vi "get_name.vi"(0 "HGF_Reference":refnum<class "HGF_Reference.lvclass">, 5 "error in (no error)":errorcluster) -> (14 "dup HGF_Reference":refnum<class "HGF_Reference.lvclass">, 16 "name":string, 19 "error out":errorcluster)   [LabVIEW 2014, in "HGF_BaseClasses.lvlib" / "HGF_Reference.lvclass"]
doc: "Get name of this reference."
uses:
  HGF_Reference.lvclass
  HGF_Reference.lvclass/HGF_Reference.ctl
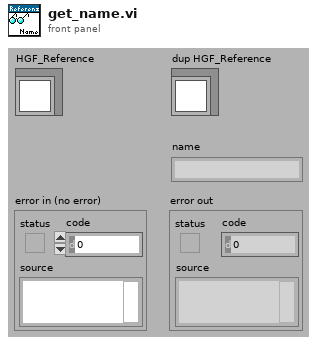
[diagram p1: front panel]
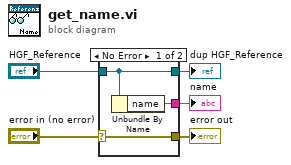
[diagram p0: block diagram]
diagram:
  n1 = case shown="No Error" "error in (no error)" {
    selector: "error in (no error)" -> [w8 w9]
    tunnel: [w8 w9] -> w4
    tunnel: [w7 w10] -> w2
    tunnel: "HGF_Reference" -> [w7 w10]
    tunnel: [w6 _] -> w1
    frame No Error {
      n2 = Unbundle By Name(w7) -> ("name"=w6:string)
    }
    frame Error {
    }
  }
  "error out" <- w4
  "dup HGF_Reference" <- w2
  "name" <- w1
